vi "2D array.vi"() -> ()   [LabVIEW 2025]
panel:
  out "Array 3":dbl[][](array[numeric])
  in  "Array 2":dbl[][](array[numeric])
  in  "Array":dbl[][](array[numeric])
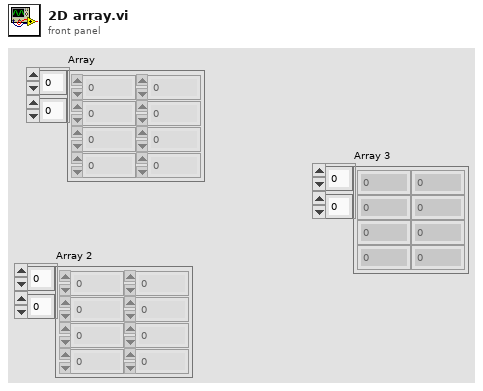
[diagram p1: front panel]
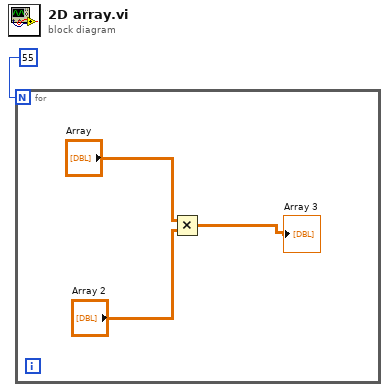
[diagram p0: block diagram]
diagram:
  n1 = for {
    N: 55 -> [_]
    n2 = Multiply(x="Array", y="Array 2") -> (x*y=→"Array 3":dbl[][])
  }
